vi "config file read-write.vi"() -> ()   [LabVIEW 2013]
uses:
  ctl/config_ctl.ctl
panel:
  in  "Config in":T1={"Trigger minlevel"=0.5, "Lower Cut-Off"=20.0, "Force high_level"=0.0, "state settings"={"method"=enum."histogram", "histogram size"=512, "histogram method"=enum."mode", "reserved"=1.0}} {"state settings"."reserved" format="%0.2f"; "Trigger minlevel" format="%#_13g"}
  out "Config out":T1={"Trigger minlevel"=0.5, "Lower Cut-Off"=20.0, "Force high_level"=0.0, "state settings"={"method"=enum."histogram", "histogram size"=512, "histogram method"=enum."mode", "reserved"=1.0}} {"state settings"."reserved" format="%0.2f"; "Trigger minlevel" format="%#_13g"}
  out "error out":errorcluster caption="에러 출력"
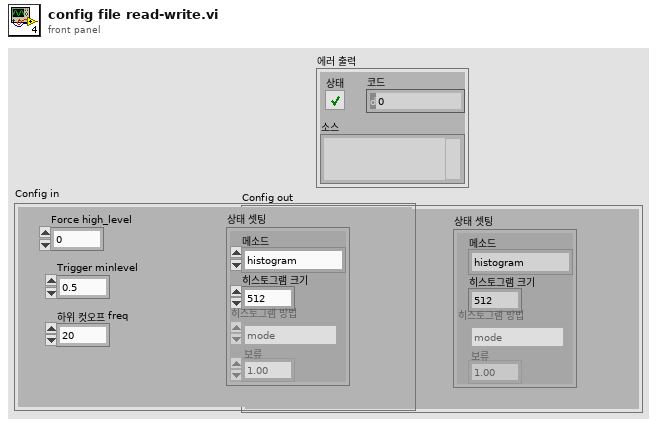
[diagram p1: front panel]
types:
  T1 = typedef "config_ctl.ctl" = cluster{"Trigger minlevel":dbl, "Lower Cut-Off":dbl, "Force high_level":dbl, "state settings":cluster{"method":enum32{"histogram", "peak", "auto select"}, "histogram size":i32, "histogram method":enum16{"mode"}, "reserved":dbl}}
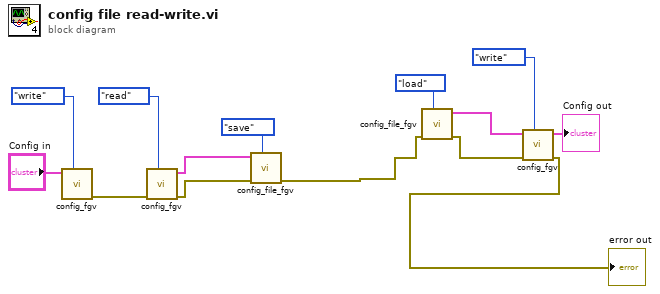
[diagram p0: block diagram]
diagram:
  n1 = call "config_fgv.vi"("cmd"=enum16{"write", "read", "ini"}."write", "Config in"="Config in") -> ("error out"=w2:errorcluster)  [unwired: 8 in, 1 out]
  n2 = call "config_fgv.vi"("cmd"=enum16{"write", "read", "ini"}."read", "error in (no error)"=w2) -> ("error out"=w4:errorcluster, "Config out"=w5:T1)  [unwired: 8 in]
  n3 = call "config_file_fgv.vi"("cmd"=enum16{"save", "load"}."save", "error in"=w4, "Config"=w5) -> ("error out"=w7:errorcluster)  [unwired: 6 in, 2 out]
  n4 = call "config_file_fgv.vi"("cmd"=enum16{"save", "load"}."load", "error in"=w7) -> ("error out"=w9:errorcluster, "var"=w8:T1)  [unwired: 7 in, 1 out]
  n5 = call "config_fgv.vi"("cmd"=enum16{"write", "read", "ini"}."write", "error in (no error)"=w9, "Config in"=w8) -> ("error out"=→"error out":errorcluster, "Config out"=→"Config out":T1)  [unwired: 7 in]
